vi "Read Plugin INI.vi"(8 "error in (no error)":errorcluster, 11 "INI file":path) -> (0 "error out":errorcluster, 3 "Plugin Details":T1={"Plugin Name"="", "Controller Type"=enum."Invalid", "Control Panel Path"=path "", "Plugin Type"=enum."Optimizer", "Config Errors"=[]})   [LabVIEW 2020, in "RxnRover.lvlib" / "Plugin Manager.lvlib"]
doc: "Reads an INI file defining a plugin to be loaded."
uses:
  Plugin Manager.lvlib
  Plugin Details.ctl
  Plugin Servers/Controller/Controller Type.ctl
  Plugin Types.ctl
  Config Error.ctl
  <vilib>/Utility/config.llb/NI_LVConfig.lvlib
  Plugin Servers/Controller/Generic Plugin.lvclass
  logging/logging.lvlib
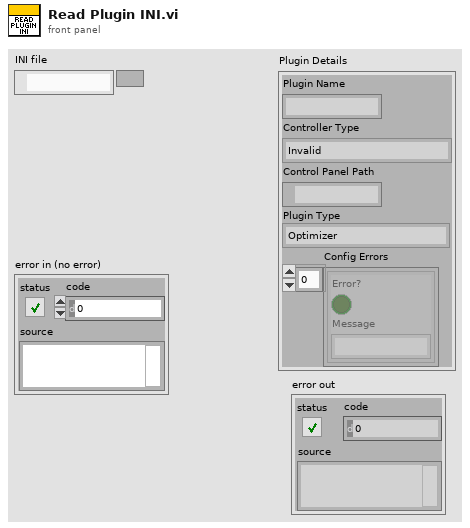
[diagram p1: front panel]
types:
  T1 = typedef "RxnRover.lvlib/Plugin Manager.lvlib/Plugin Details.ctl" = cluster{"Plugin Name":string, "Controller Type":T2, "Control Panel Path":path, "Plugin Type":T3, "Config Errors":T4[]}
  T2 = typedef "RxnRover.lvlib/Generic Plugin.lvclass/Controller Type.ctl" = enum16{"Invalid", "Temperature Controller", "Pump Controller", "Syringe Pump", "Generic Optimizer", "LC Parser", "Passive Hardware"}
  T3 = typedef "RxnRover.lvlib/Plugin Manager.lvlib/Plugin Types.ctl" = enum16{"Invalid", "Optimizer", "Analyzer", "Hardware"}
  T4 = typedef "RxnRover.lvlib/Plugin Manager.lvlib/Config Error.ctl" = cluster{"Error?":bool, "Message":string}
  T5 = typedef "NI_LVConfig.lvlib/Config Data RefNum.ctl" = refnum<k1>
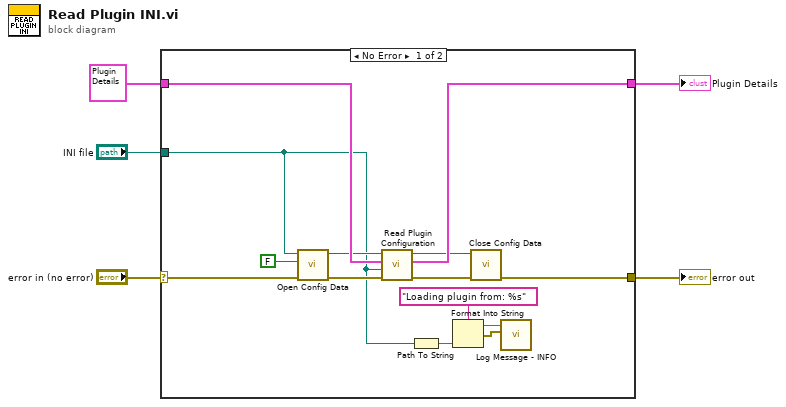
[diagram p0: block diagram]
diagram:
  n1 = case shown="No Error" "error in (no error)" {
    selector: "error in (no error)" -> [w19 w21]
    tunnel: [w15 w21] -> w4
    tunnel: "INI file" -> [w6 _]
    tunnel: T1 {"Plugin Name"="", "Controller Type"=enum."Invalid", "Control Panel Path"=path "", "Plugin Type"=enum."Optimizer", "Config Errors"=[]} ("Plugin Details") -> [w12 w20]
    tunnel: [w16 w20] -> w1
    frame No Error {
      n2 = call <vilib>:"Open Config Data.vi"("error in (no error)"=w19, "create file if necessary (T)"=FALSE, "configuration file path"=w6) -> ("error out"=w13:errorcluster, "refnum"=w11:T5)  [unwired: 6 in, 1 out]
      n3 = call "Read Plugin Configuration.vi"("error in (no error)"=w13, "Plugin File Path"=w6, "Plugin Details in"=w12, "Refnum in"=w11) -> ("error out"=w18:errorcluster, "Plugin Details out"=w16:T1, "refnum out"=w14:T5)  [unwired: 5 in]
      n4 = Path To String(path=w6) -> (string=w7:string)
      n5 = Format Into String(format string="Loading plugin from: %s", w7) -> (resulting string=w9:string, error out=w10:errorcluster)  [unwired: 2 in]
      n6 = call <vilib>:"Close Config Data.vi"("error in (no error)"=w18, "refnum"=w14) -> ("error out"=w15:errorcluster)  [unwired: 8 in, 1 out]
      n7 = call "Log Message - INFO.vi"("error in (no error)"=w10, "Message"=w9) -> ()  [unwired: 9 in, 1 out]
    }
    frame Error {
    }
  }
  "error out" <- w4
  "Plugin Details" <- w1
